vi "Destroy Front Panel Events.vi"(8 "error in":errorcluster, 11 "Main Window in":refnum<class "Main Window.lvclass">) -> (0 "error out":errorcluster, 3 "Main Window out":refnum<class "Main Window.lvclass">)   [LabVIEW 2023, in "Main Window.lvlib" / "Main Window.lvclass"]
uses:
  Main Window.lvclass
  Main Window.lvclass/Main Window.ctl
  UI Window/UI Window.lvclass
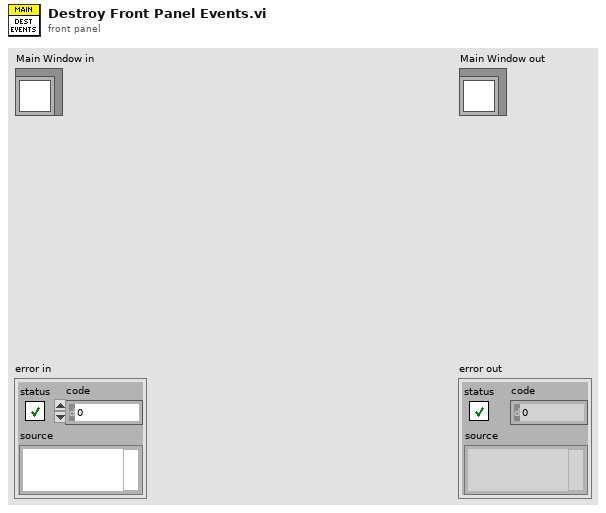
[diagram p1: front panel]
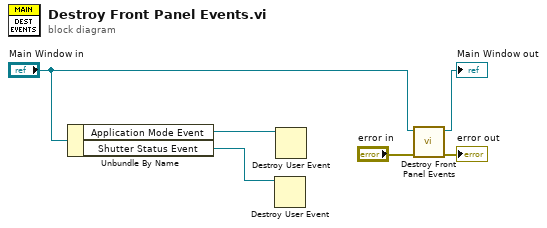
[diagram p0: block diagram]
diagram:
  n1 = Unbundle By Name("Main Window in") -> ("Application Mode Event"=w3:refnum<user-event>, "Shutter Status Event"=w1:refnum<user-event>)
  n2 = Destroy User Event(user event=w1) -> ()  [unwired: 1 in, 1 out]
  n3 = Destroy User Event(user event=w3) -> ()  [unwired: 1 in, 1 out]
  n4 = call-parent "Destroy Front Panel Events.vi"("error in (no error)"="error in", "UI Window in"="Main Window in") -> ("error out"=→"error out":errorcluster, "UI Window out"=→"Main Window out":refnum<class "Main Window.lvclass">)  [unwired: 8 in]
